vi "SRV_Command Queue Error-State Controller.vi"(7 "Filter Error Codes (empty)":i32[](array[numeric]), 8 "error in (no error)":errorcluster, 10 "Error Command":string="Error", 11 "Command-Data Queue":refnum<queue>) -> (0 "error out":errorcluster, 3 "Command-Data Queue out":refnum<queue>)   [LabVIEW 2009]
doc: "This VI is used to control state transition in the case of an input error. If \"error in\" contains an error, the error is compared with the Filter Error Codes array. If the error is found in the Filter Error Codes array, the error is stripped and the no new states are added to the state queue. If the error code is not filtered, the state queue is populated with the command from the \"Error Command\" input and \"Data\" set to the error cluster.\n\n<B>If the Error Command input is unwired or if you input an empty string, then it inserts \"Error\" on the queue.</B>\n\n\nAuthor: Mike Schultz\n\n\nLogicPD, Inc\nwww.logicpd.com"
uses:
  SRV_Command-Data Queue Data Type.ctl
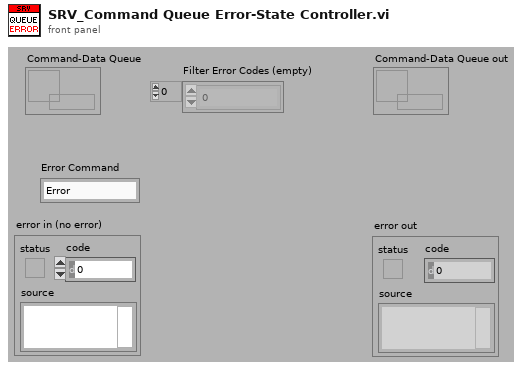
[diagram p1: front panel]
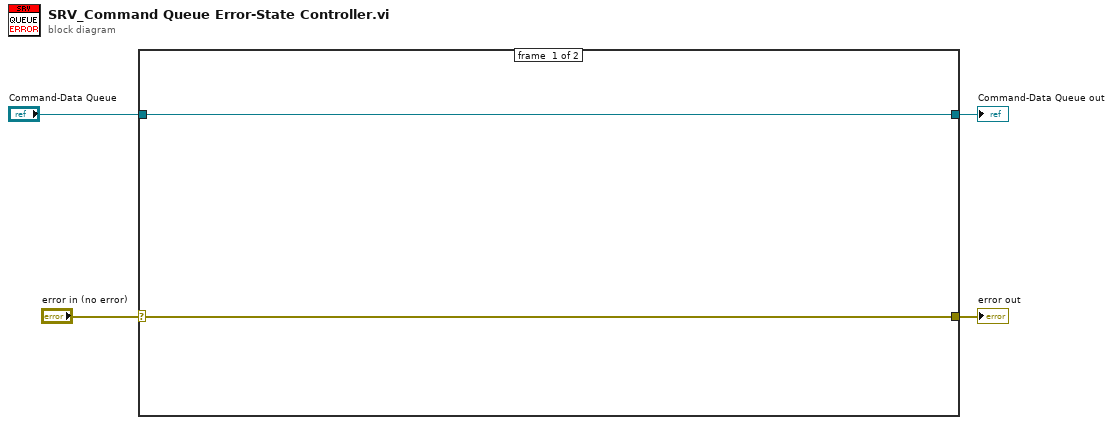
[diagram p0: block diagram]
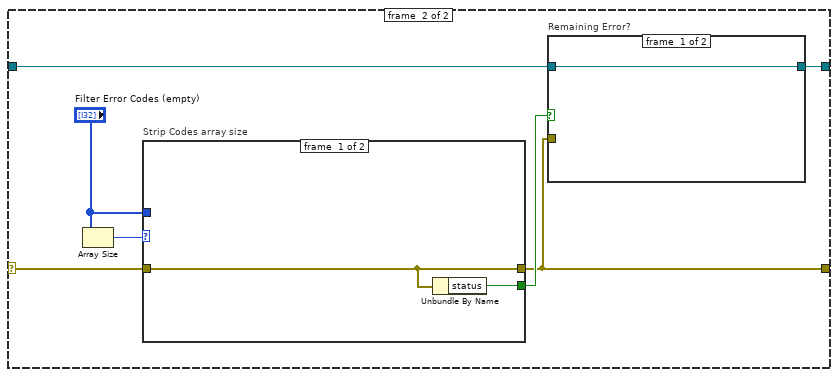
[diagram p2: hidden frame]
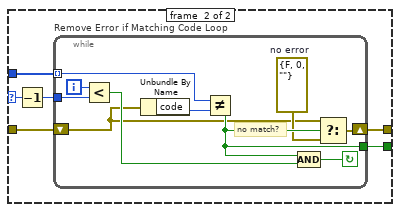
[diagram p3: hidden frame]
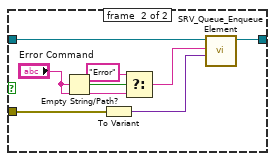
[diagram p4: hidden frame]
diagram:
  n1 = case "Error In?" shown="Error" "error in (no error)" {
    selector: "error in (no error)" -> [w5 w10]
    tunnel: [w5 w7] -> w4
    tunnel: "Command-Data Queue" -> [w6 w13]
    tunnel: [w6 w12] -> w1
    frame #0 {
    }
    frame #1 {
      n2 = Array Size(array="Filter Error Codes (empty)") -> (size(s)=w8:i32)
      n3 = case "Strip Codes array size" shown="1.." w8 {
        selector: w8 -> [_ w16]
        tunnel: "Filter Error Codes (empty)" -> [_ w21]
        tunnel: w10 -> [w15 w20]
        tunnel: [w15 w19] -> w7
        tunnel: [w14 w17] -> w9
        frame #0 {
          n4 = Unbundle By Name(w15) -> ("status"=w14:bool)
        }
        frame #1 {
          n5 = Decrement(x=w16) -> (x-1=w18:i32)
          n6 = while "Remove Error if Matching Code Loop" {
            tunnel: [w24] -> w17
            tunnel: w18 -> [w28]
            shift-left: w20 -> [w22]
            shift-right: [w25] -> w19
            tunnel: w21 -> [w27] mode=indexing
            i -> [w29]
            stop <- w31 continue-if-true
            w23 = errorcluster {"status"=FALSE, "code"=0, "source"=""}  # no error
            # "no match?"
            n7 = Less?(x=w29, y=w28) -> (x < y?=w30:bool)
            n8 = Unbundle By Name(w22) -> ("code"=w26:i32)
            n9 = Not Equal?(x=w27, y=w26) -> (x != y?=w24:bool)
            n10 = Compound Arithmetic op=AND(w24, w30) -> (w31:bool)
            n11 = Select(t=w22, s=w24, f=w23) -> (s? t:f=w25:errorcluster)
          }
        }
      }
      n12 = case "Remaining Error?" shown="True" w9 {
        tunnel: w13 -> [w32 w39]
        tunnel: [w32 w40] -> w12
        tunnel: w7 -> [_ w34]
        frame #0 {
        }
        frame #1 {
          n13 = Empty String/Path?(string/path="Error Command") -> (empty?=w38:bool)
          n14 = To Variant(anything=w34) -> (Variant=w33:variant)
          n15 = Select(t="Error" ("Error Command"), s=w38, f="Error Command") -> (s? t:f=w35:string)
          n16 = call "SRV_Queue_Enqueue Element.vi"("Data"=w33, "Command"=w35, "Command-Data Queue"=w39) -> ("Command-Data Queue out"=w40:refnum<queue>)  [unwired: 6 in, 2 out]
        }
      }
    }
  }
  "error out" <- w4
  "Command-Data Queue out" <- w1
